vi "V7310.Main.vi"() -> ()   [LabVIEW 2016]
uses:
  V7310.Data.ctl
  V7310.Data.Status.ctl
  V7310.Data.Status.State.ctl
  LowLevel/V7310.LaserStatus.ctl
  LowLevel/V7310.Message.Data.ctl
  LowLevel/V7310.Job.Variable.ctl
  V7310.Data.Sets.ctl
  V7310.Action.ctl
  tools/CitTemplate/citTemplate.errData.ctl
  tools/EventLog/EventLog.EventSource.ctl
  LowLevel/V7310.Job.Data.ctl
  LowLevel/V7310.Job.Sets.ctl
  Global/ApplicationGlobal.vi
  LowLevel/V7310.Global.vi
panel:
  out "Action":T1=enum."--- V7310 ---"
  out "Data":T2={"Status"={"State"=enum."Init", "LaserStatus"=enum."-", "LaserStatusRaw"="", "Ref"=refnum, "RTC TS"=timestamp(0 s since 1904-01-01), "Conn TS"=timestamp(0 s since 1904-01-01), "Msg"=[], "JobInUse"="", "Jobs"=[], "Vars"=[]}, "Sets"={"Address"="192.168.2.1", "Timeout_ms"=5000, "ReconnectPeriod_s"=0, "JobInUse"="", "CoordinatesOffset"={"X"=0.0, "Y"=0.0}}}
  out "_loop":i32(ring)=4
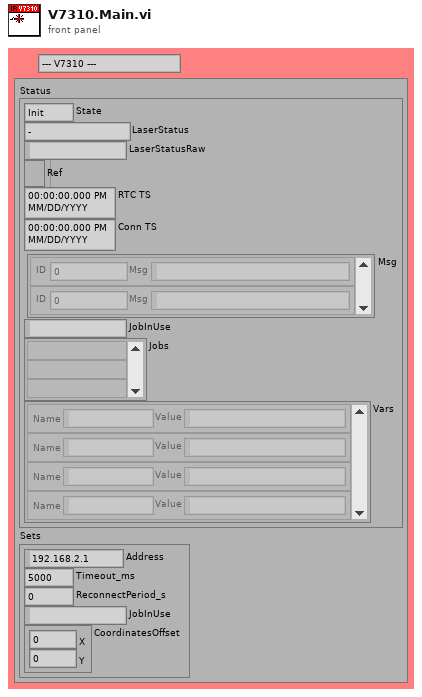
[diagram p1: front panel]
types:
  T1 = typedef "V7310.Action.ctl" = enum32{"idle", "constructor", "destructor", "--- V7310 ---", "Init", "Select", "Start", "Stop"}
  T2 = typedef "V7310.Data.ctl" = cluster{"Status":T3, "Sets":T8}
  T3 = typedef "V7310.Data.Status.ctl" = cluster{"State":T4, "LaserStatus":T5, "LaserStatusRaw":string, "Ref":refnum<k5>, "RTC TS":timestamp, "Conn TS":timestamp, "Msg":T6[], "JobInUse":string, "Jobs":string[], "Vars":T7[]}
  T4 = typedef "V7310.Data.Status.State.ctl" = enum16{"First", "Init", "Msg", "Error", "Abort", "Idle", "Run"}
  T5 = typedef "V7310.LaserStatus.ctl" = enum16{"-", "FatalError", "Initialize", "KeySwitchOpen", "TimeoutInterlock", "InterlockOpen", "StartUp", "ShutterlockOpen", "Standby", "Ready", "PrepareForMarking", "WaitForTrigger", "Marking"}
  T6 = typedef "V7310.Message.Data.ctl" = cluster{"ID":i32, "Msg":string}
  T7 = typedef "V7310.Job.Variable.ctl" = cluster{"Name":string, "Value":string}
  T8 = typedef "V7310.Data.Sets.ctl" = cluster{"Address":string, "Timeout_ms":i32, "ReconnectPeriod_s":i32, "JobInUse":string, "CoordinatesOffset":cluster{"X":dbl, "Y":dbl}}
  T9 = typedef "citTemplate.errData.ctl" = cluster{"ts":timestamp, "src":T10, "instance":i32, "action":string, "error":errorcluster, "unconfirmed":bool}
  T10 = typedef "EventLog.EventSource.ctl" = enum16{"All", "Gui", "Ref", "File", "Arch", "Seq", "CPX", "DB", "Laser", "Scan.P", "Scan.O"}
  T11 = typedef "V7310.Job.Data.ctl" = cluster{"Vars":string[], "Sets":T12}
  T12 = typedef "V7310.Job.Sets.ctl" = cluster{"X":dbl, "Y":dbl, "Angle":dbl}
  T13 = typedef "citTemplate.notifierHandle.ctl" = refnum<notifier>
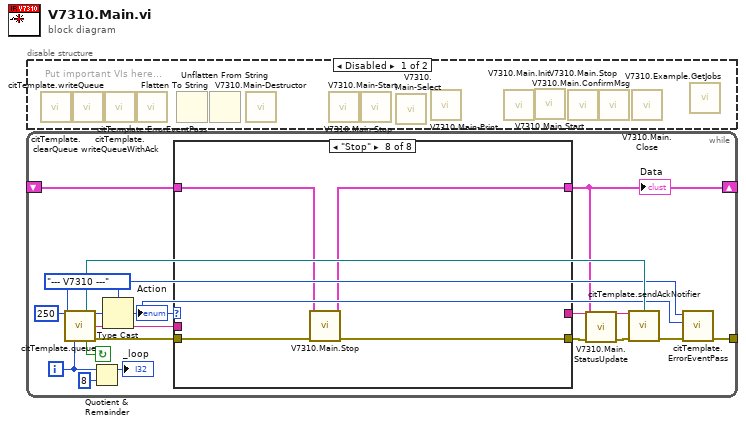
[diagram p0: block diagram]
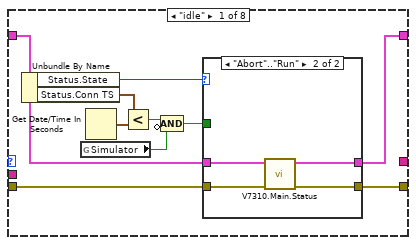
[diagram p3: hidden frame]
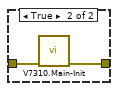
[diagram p5: hidden frame]
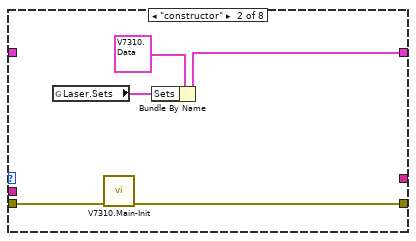
[diagram p6: hidden frame]
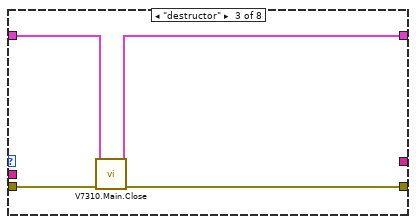
[diagram p7: hidden frame]
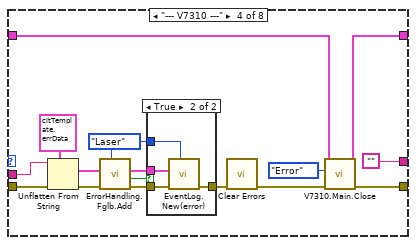
[diagram p8: hidden frame]
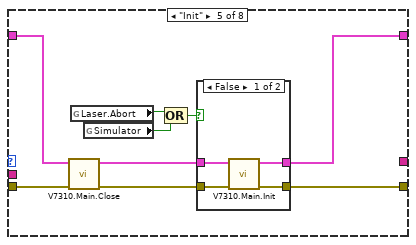
[diagram p10: hidden frame]
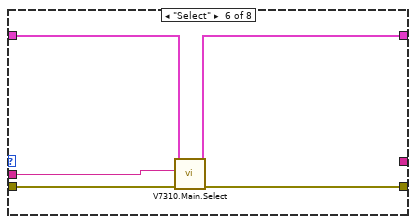
[diagram p12: hidden frame]
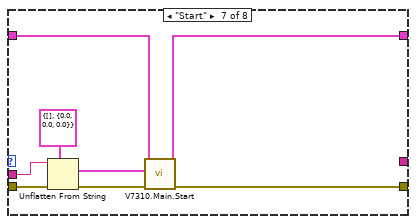
[diagram p13: hidden frame]
diagram:
  n1 = while {
    tunnel: [w8] -> _
    shift-right: [w1] -> _
    shift-left: _ -> [w5]
    i -> [w4]
    stop <- w15 continue-if-true
    w12 = V7310.Action."--- V7310 ---" ("Action")
    n2 = call "citTemplate.queue.vi"("ms timeout (250 ms)"=250, "event enum"=w12, "iteration (-1)"=w4) -> ("notifierHandle out"=w14:T13, "event out"=w17:u32, "(flatten) data out"=w16:string, "continue"=w15:bool, "error out"=w6:errorcluster)  [unwired: 2 in, 6 out]
    n3 = Quotient & Remainder(x=w4, y=8) -> (x-y*floor(x/y)=→"_loop":i32)  [unwired: 1 out]
    n4 = Type Cast(type=w12, x=w17) -> (*(type *) &x=w9:T1)
    "Action" <- w9
    n5 = case shown="\"Stop\"" w9 {
      tunnel: w16 -> [_ _ _ w61 _ w83 w90 _]
      tunnel: [_ _ _ "" _ _ _ _] -> w13
      tunnel: [w26 w42 w46 w52 w76 w87 w95 w99] -> w2
      tunnel: w6 -> [w27 w43 w47 w60 w75 w84 w92 w96]
      tunnel: w5 -> [w24 _ w45 w51 w73 w85 w93 w97]
      tunnel: [w23 w39 w44 w50 w71 w86 w94 w98] -> w1
      frame "idle" {
        n6 = Unbundle By Name(w24) -> ("Status.State"=w25:T4, "Status.Conn TS"=w19:timestamp)
        n7 = global read "ApplicationGlobal.vi" "Simulator"() -> (w20:bool)
        n8 = Get Date/Time In Seconds() -> (seconds since 1Jan1904=w22:timestamp)
        n9 = Less?(x=w19, y=w22) -> (x < y?=w21:bool)
        n10 = Compound Arithmetic op=AND(w21, invert w20) -> (w18:bool)
        n11 = case shown="\"Abort\"..\"Run\"" w25 {
          tunnel: w27 -> [w29 w38]
          tunnel: [w31 w35] -> w26
          tunnel: [w30 w37] -> w23
          tunnel: w24 -> [w30 w36]
          tunnel: w18 -> [w28 _]
          frame Default {
            n12 = case shown="False" w28 {
              tunnel: [w32 w33] -> w31
              tunnel: w29 -> [w32 w34]
              frame False {
              }
              frame True {
                n13 = call "V7310.Main-Init.vi"("error in"=w34) -> ("error out"=w33:errorcluster)  [unwired: 10 in]
              }
            }
          }
          frame "Abort".."Run" {
            n14 = call "V7310.Main.Status.vi"("error in"=w38, "Data in"=w36) -> ("error out"=w35:errorcluster, "Data out"=w37:T2)  [unwired: 8 in]
          }
        }
      }
      frame "constructor" {
        n15 = global read "V7310.Global.vi" "Laser.Sets"() -> (w41:T8)
        n16 = call "V7310.Main-Init.vi"("error in"=w43) -> ("error out"=w42:errorcluster)  [unwired: 10 in]
        n17 = Bundle By Name(cluster=T2 {"Status"={"State"=enum."First", "LaserStatus"=enum."-", "LaserStatusRaw"="", "Ref"=refnum, "RTC TS"=timestamp(0 s since 1904-01-01), "Conn TS"=timestamp(0 s since 1904-01-01), "Msg"=[], "JobInUse"="", "Jobs"=[], "Vars"=[]}, "Sets"={"Address"="", "Timeout_ms"=0, "ReconnectPeriod_s"=0, "JobInUse"="", "CoordinatesOffset"={"X"=0.0, "Y"=0.0}}} ("Data"), "Sets"=w41) -> (w39:T2)
      }
      frame "destructor" {
        n18 = call "V7310.Main.Close.vi"("error in"=w47, "Data in"=w45) -> ("error out"=w46:errorcluster, "Data out"=w44:T2)  [unwired: 8 in]
      }
      frame "--- V7310 ---" {
        w56 = EventLog.EventSource."Laser" ("Event source")
        n19 = Unflatten From String(type=T9 {"ts"=timestamp(0 s since 1904-01-01), "src"=enum."All", "instance"=0, "action"="", "error"={"status"=FALSE, "code"=0, "source"=""}, "unconfirmed"=FALSE} ("ErrData"), binary string=w61, error in (no error)=w60) -> (value=w55:T9, error out=w54:errorcluster)  [unwired: 3 out]
        n20 = call "ErrorHandling.Fglb.Add.vi"("Event source"=w56, "error in (no error)"=w54, "Error in"=w55) -> ("error out"=w58:errorcluster, "changed?"=w48:bool)  [unwired: 7 in]
        n21 = case shown="True" w48 {
          tunnel: w58 -> [w63 w67]
          tunnel: [w63 w66] -> w57
          tunnel: w56 -> [_ w65]
          tunnel: w55 -> [_ w64]
          frame False {
          }
          frame True {
            n22 = call "EventLog.New(error).vi"("Source (All)"=w65, "error in"=w67, "ErrData"=w64) -> ("error out"=w66:errorcluster)  [unwired: 8 in]
          }
        }
        n23 = call <vilib>:"Clear Errors.vi"("error in (no error)"=w57) -> ("error out"=w53:errorcluster)  [unwired: 5 in, 1 out]
        n24 = call "V7310.Main.Close.vi"("error in"=w53, "State (Init)"=V7310.Data.Status.State."Error", "Data in"=w51) -> ("error out"=w52:errorcluster, "Data out"=w50:T2)  [unwired: 7 in]
      }
      frame "Init" {
        n25 = call "V7310.Main.Close.vi"("error in"=w75, "Data in"=w73) -> ("error out"=w74:errorcluster, "Data out"=w72:T2)  [unwired: 8 in]
        n26 = global read "V7310.Global.vi" "Laser.Abort"() -> (w70:bool)
        n27 = global read "ApplicationGlobal.vi" "Simulator"() -> (w68:bool)
        n28 = Compound Arithmetic op=OR(w70, w68) -> (w69:bool)
        n29 = case shown="False" w69 {
          tunnel: [w80 w81] -> w76
          tunnel: w74 -> [w79 w81]
          tunnel: w72 -> [w78 w82]
          tunnel: [w77 w82] -> w71
          frame False {
            n30 = call "V7310.Main.Init.vi"("error in"=w79, "Data in"=w78) -> ("error out"=w80:errorcluster, "Data out"=w77:T2)  [unwired: 8 in]
          }
          frame True {
          }
        }
      }
      frame "Select" {
        n31 = call "V7310.Main.Select.vi"("error in"=w84, "Job"=w83, "Data in"=w85) -> ("error out"=w87:errorcluster, "Data out"=w86:T2)  [unwired: 7 in]
      }
      frame "Start" {
        n32 = Unflatten From String(type=T11 {"Vars"=[], "Sets"={"X"=0.0, "Y"=0.0, "Angle"=0.0}}, binary string=w90, error in (no error)=w92) -> (value=w89:T11, error out=w91:errorcluster)  [unwired: 2 in, 1 out]
        n33 = call "V7310.Main.Start.vi"("error in"=w91, "Job"=w89, "Data in"=w93) -> ("error out"=w95:errorcluster, "Data out"=w94:T2)  [unwired: 7 in]
      }
      frame "Stop" {
        n34 = call "V7310.Main.Stop.vi"("error in"=w96, "Data in"=w97) -> ("error out"=w99:errorcluster, "Data out"=w98:T2)  [unwired: 8 in]
      }
    }
    "Data" <- w1
    n35 = call "V7310.Main.StatusUpdate.vi"("error in"=w2, "Data in"=w1) -> ("error out"=w3:errorcluster)  [unwired: 9 in]
    n36 = call "citTemplate.sendAckNotifier.vi"("notification data"=w13, "notifierHandle in"=w14, "error in"=w3) -> ()  [unwired: 13 out]
    n37 = call "citTemplate.ErrorEventPass.vi"("error in"=w3, "action of error"=w9, "event in"=w12) -> ("error out"=w8:errorcluster)  [unwired: 2 in, 6 out]
  }
  n38 = disable-structure shown="Disabled" {
    frame Disabled {
      # "Put important VIs here..."
      n39 = call "citTemplate.clearQueue.vi"() -> ()  [unwired: 14 in, 2 out]
      n40 = call "citTemplate.writeQueue.vi"() -> ()  [unwired: 15 in, 1 out]
      n41 = call "citTemplate.writeQueueWithAck.vi"() -> ()  [unwired: 13 in, 3 out]
      n42 = call "citTemplate.ErrorEventPass.vi"() -> ()  [unwired: 11 in, 1 out]
      n43 = Flatten To String() -> ()  [unwired: 4 in, 3 out]
      n44 = Unflatten From String() -> ()  [unwired: 5 in, 3 out]
      n45 = call "V7310.Main-Destructor.vi"() -> ()  [unwired: 11 in, 1 out]
      n46 = call "V7310.Main-Start.vi"() -> ()  [unwired: 10 in, 2 out]
      n47 = call "V7310.Main-Stop.vi"() -> ()  [unwired: 11 in, 1 out]
      n48 = call "V7310.Main-Select.vi"() -> ()  [unwired: 10 in, 2 out]
      n49 = call "V7310.Main-Print.vi"() -> ()  [unwired: 7 in, 5 out]
      n50 = call "V7310.Main.Init.vi"() -> ()  [unwired: 10 in, 2 out]
      n51 = call "V7310.Main.Start.vi"() -> ()  [unwired: 10 in, 2 out]
      n52 = call "V7310.Main.Stop.vi"() -> ()  [unwired: 10 in, 2 out]
      n53 = call "V7310.Main.ConfirmMsg.vi"() -> ()  [unwired: 10 in, 2 out]
      n54 = call "V7310.Main.Close.vi"() -> ()  [unwired: 10 in, 2 out]
      n55 = call "V7310.Example.GetJobs.vi"() -> ()  [unwired: 12 in]
    }
    frame Enabled {
    }
  }
